vi "Controller Global.vi"(8 "error in (no error)":errorcluster, 9 "Control In":T1={"I-O.lvclass"=refnum, "Gantry"=refnum, "Dispenser"="COM1"}, 10 "Action":enum16{"Initialize", "Read", "Write"}(ring)=enum."Write", 11 "Assembly Run in":refnum<class "Assembly Run.lvclass">) -> (0 "error out":errorcluster, 2 "Control Out":T1={"I-O.lvclass"=refnum, "Gantry"=refnum, "Dispenser"="COM1"}, 3 "Assembly Run out":refnum<class "Assembly Run.lvclass">)   [LabVIEW 2020, in "Assembly Run.lvclass"]
uses:
  Assembly Run.lvclass
  Controller/Controller.lvclass
  Controller/I-O/I-O.lvclass
  Controller/Controllers.ctl
  C:/Program Files (x86)/Aerotech/A3200/LabVIEW/2010/Bin/Aerotech.A3200.dll
  Program Files (x86)/Aerotech/A3200/LabVIEW/2010/Bin/Aerotech.A3200.dll
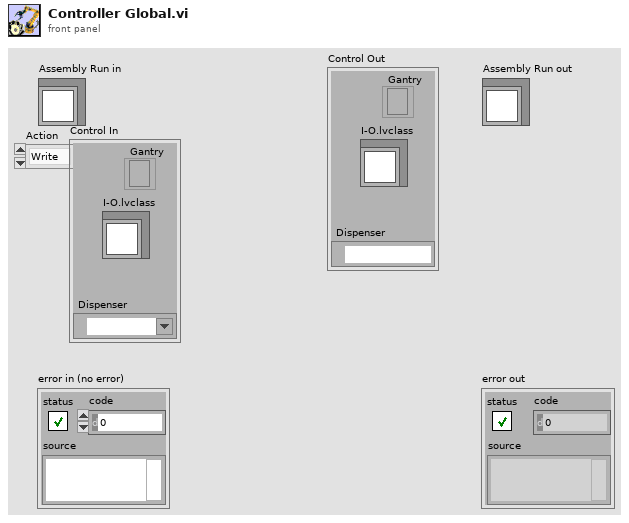
[diagram p1: front panel]
types:
  T1 = typedef "Controller.lvclass/Controllers.ctl" = cluster{"I-O.lvclass":refnum<class "I-O.lvclass">, "Gantry":refnum<k24>, "Dispenser":refnum<visa-resource-name>}
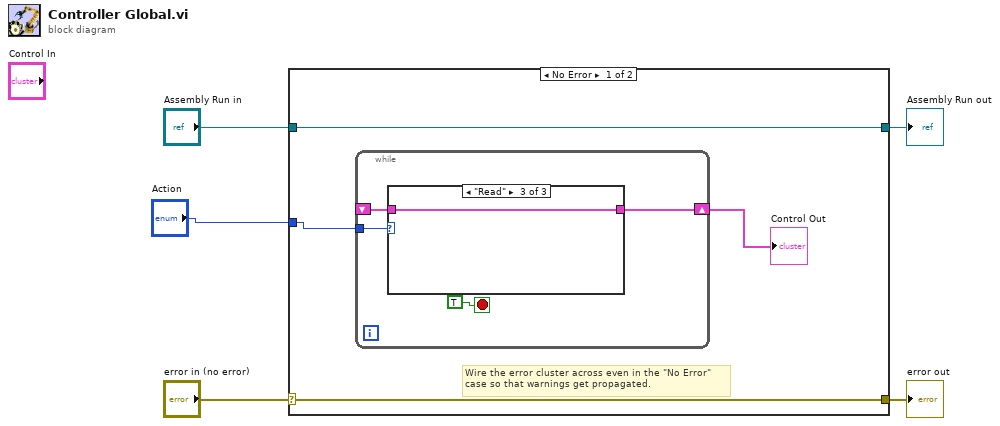
[diagram p0: block diagram]
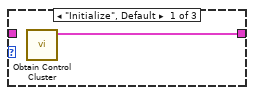
[diagram p2: hidden frame]
diagram:
  n1 = case shown="No Error" "error in (no error)" {
    selector: "error in (no error)" -> [w8 w18]
    tunnel: [w8 w18] -> w4
    tunnel: [w9 w17] -> w2
    tunnel: "Assembly Run in" -> [w9 w17]
    tunnel: "Action" -> [w7 _]
    frame No Error {
      # "Wire the error cluster across even in the \"No Error\"\ncase so that warnings get propagated."
      n2 = while {
        tunnel: w7 -> [w13]
        shift-right: [w11] -> w6
        shift-left: _ -> [w10]
        stop <- TRUE stop-if-true
        n3 = case shown="\"Read\"" w13 {
          tunnel: [w14 w15 w16] -> w11
          tunnel: w10 -> [_ w15 w16]
          frame "Initialize", Default {
            n4 = call "Obtain Control Cluster.vi"() -> ("Control Out"=w14:T1)  [unwired: 11 in]
          }
          frame "Write" {
          }
          frame "Read" {
          }
        }
      }
      "Control Out" <- w6
    }
    frame Error {
    }
  }
  "error out" <- w4
  "Assembly Run out" <- w2
